vi "SimpleDemo old.vi"() -> ()   [LabVIEW 2011]
uses:
  C:/Users/Behavior Room/Desktop/Kinect Mouse/DepthSense/FunctionPointerProxy/FunctionPointerProxy/obj/Release/FunctionPointerProxy.dll
  FunctionPointerProxy/obj/Release/FunctionPointerProxy.dll
  <vilib>/vision/Image Controls.llb/IMAQ Image.ctl
  <vilib>/Platform/TimedLoop/XDataNode/timing_clust.ctl
  <vilib>/Platform/TimedLoop/XDataNode/nitl_modes.ctl
  <vilib>/Platform/TimedLoop/XDataNode/wakeup.ctl
  <vilib>/Platform/TimedLoop/XDataNode/XDataNode.xnode
  <userlib>/libOptrima-2-3/libOptrima-2-3.lvlib
  <vilib>/Platform/TimedLoop/XDataNode/XDNodeRunTimeDep.lvlib
  Program Files (x86)/SoftKinetic/OptrimaSDK/lib/libOptrima-2-3.dll
panel:
  out "length":i32
  out "add newframe\ncallback":i32
  in  "stop":bool
  in  "Buffer Size 3":i32=10
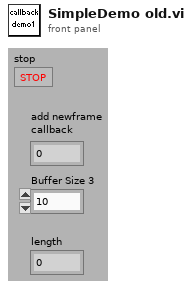
[diagram p1: front panel]
types:
  T1 = typedef "IMAQ Image.ctl" = refnum<image>
  T2 = typedef "XDNodeRunTimeDep.lvlib/timing_clust.ctl" = cluster{"Expected End [f-1]":u64, "Actual End [f-1]":u64, "Finished Late? [f-1]":bool, "Expected End [i-1]":u64, "Actual End [i-1]":u64, "Finished Late? [i-1]":bool, "Expected Start [i]":u64, "Actual Start [i]":u64, "Expected Start [f]":u64, "Actual Start [f]":u64, "Source Name":string, "Structure Name":string, "Period":i64, "Deadline":i64, "Offset":i64, "Start":i64, "Priority":i32, "Timeout":i32, "Mode":T3, "Wakeup Reason":T4, "Error":errorcluster, "Source Type":string, "Secondary Source Type":string, "Global End Time":u64, "Global Start Time":u64, "Frame Duration":u64, "Iteration Duration":u64, "Assigned CPU":i32, "I/O Scan Engine Mode":u32}
  T3 = typedef "XDNodeRunTimeDep.lvlib/nitl_modes.ctl" = enum32{"No Change", "Process missed periods, maintain original phase", "Discard missed periods, maintain original phase", "Process missed periods, ignore original phase", "Discard missed periods, ignore original phase"}
  T4 = typedef "XDNodeRunTimeDep.lvlib/wakeup.ctl" = enum32{"Normal", "Aborted", "Asynchronous wakeup", "Timing source error", "Timed loop error", "Timeout"}
  T5 = cluster{"queue out":refnum<queue>, "queue out":refnum<queue>}
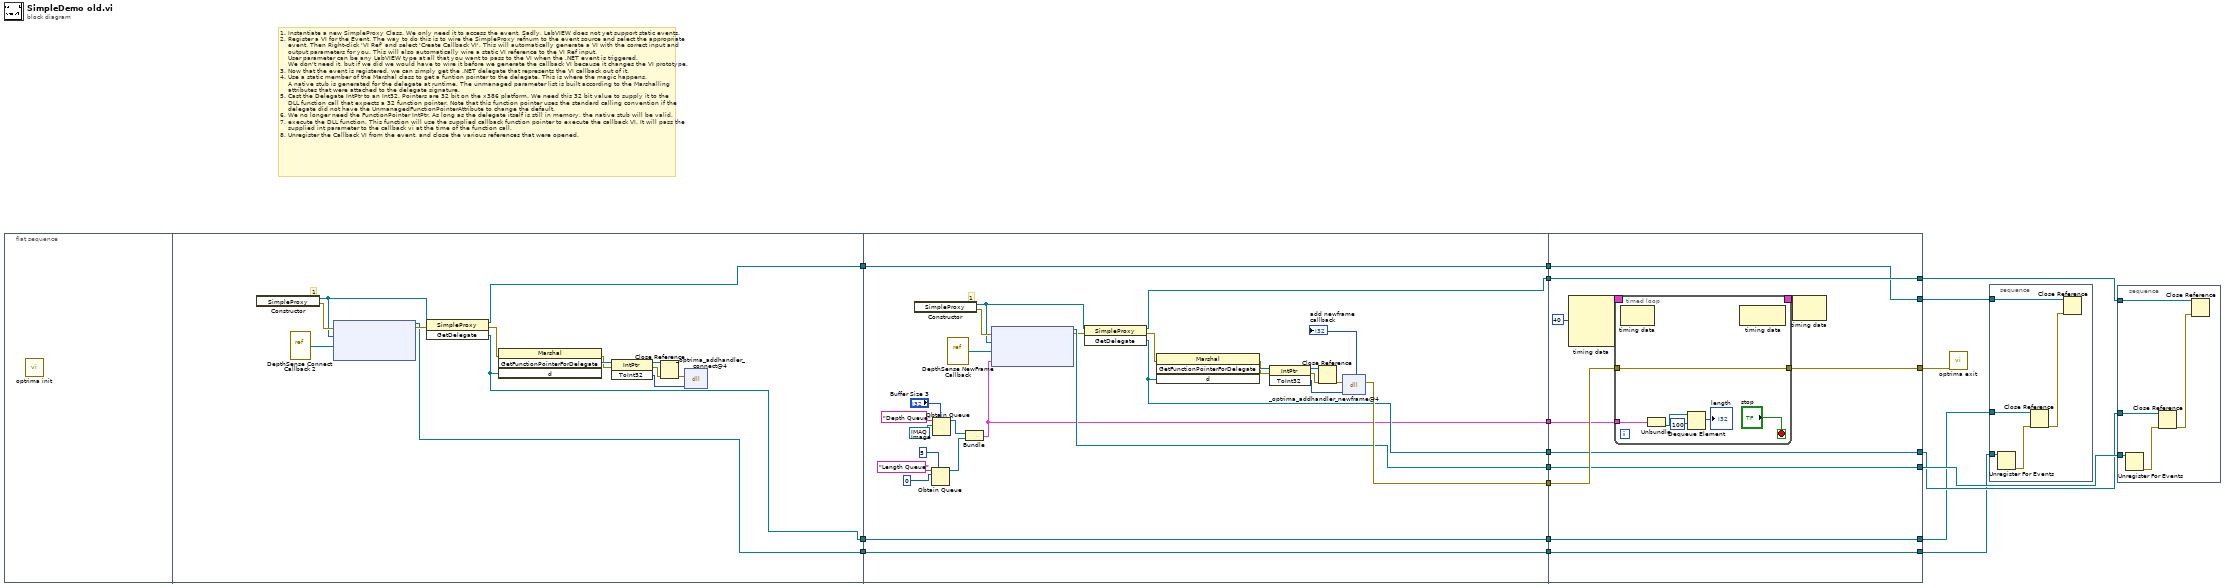
[diagram p0: block diagram]
diagram:
  # "1. Instantiate a new SimpleProxy Class. We only need it to access the event. Sadly, LabVIEW does not yet support static events.\n2. Register a VI for the Event. The way to do this is to wire the SimpleProxy refnum to the event source and select the appropriate\n    event. Then Right-click 'VI Ref' and select 'Create Callback VI'. This will automatically generate a VI with the correct input and\n    output parameters for you. This will also automatically wire a static VI reference to the VI Ref input.\n    User parameter can be any LabVIEW type at all that you want to pass to the VI when the .NET event is triggered.\n    We don't need it, but if we did we would have to wire it before we generate the callback VI because it changes the VI prototype.\n3. Now that the event is registered, we can simply get the .NET delegate that represents the VI callback out of it.\n4. Use a static member of the Marshal class to get a funtion pointer to the delegate. This is where the magic happens.\n    A native stub is generated for the delegate at runtime. The unmanaged parameter list is built according to the Marshalling\n    attributes that were attached to the delegate signature.\n5. Cast the Delegate IntPtr to an Int32. Pointers are 32 bit on the x386 platform. We need this 32 bit value to supply it to the\n    DLL function call that expects a 32 function pointer. Note that this function pointer uses the standard calling convention if the\n    delegate did not have the UnmanagedFunctionPointerAttribute to change the default.\n6. We no longer need the FunctionPointer IntPtr. As long as the delegate itself is still in memory, the native stub will be valid.\n7. execute the DLL function. This function will use the supplied callback function pointer to execute the callback VI. It will pass the\n    supplied int parameter to the callback vi at the time of the function call.\n8. Unregister the Callback VI from the event, and close the various references that were opened."
  n1 = flat-sequence {
    tunnel: [w21] -> w9
    tunnel: [w20] -> w6
    tunnel: [w19] -> w3
    tunnel: [w60] -> w18
    tunnel: [w59] -> w16
    tunnel: [w58] -> w14
    tunnel: [w57] -> w11
    tunnel: [w56] -> w10
    tunnel: w9 -> [w56]
    tunnel: w6 -> [w55]
    tunnel: [w55] -> w5
    tunnel: [w54] -> w4
    tunnel: w3 -> [w54]
    tunnel: [w34] -> w1
    tunnel: w18 -> [w72]
    tunnel: [w71] -> w17
    tunnel: [w67] -> w15
    tunnel: w16 -> [w67]
    tunnel: [w66] -> w13
    tunnel: w14 -> [w66]
    tunnel: [w65] -> w12
    tunnel: w11 -> [w65]
    tunnel: w10 -> [w64]
    tunnel: [w64] -> w8
    tunnel: [w63] -> w7
    tunnel: w5 -> [w63]
    tunnel: w4 -> [w62]
    tunnel: [w62] -> w2
    tunnel: w1 -> [w61]
    frame #0 {
      n2 = call <userlib>:"optrima init.vi"() -> ()  [unwired: 11 in, 1 out]
    }
    frame #1 {
      # "1"
      n3 = constructor class="SimpleProxy"() -> (reference out=w24:refnum<k24>, error out=w28:errorcluster)  [unwired: 3 in, 1 out]
      n4 = vi-ref "DepthSense Connect Callback 2.vi"() -> ("vi reference"=w22:refnum<vi>)
      n5 = node(w28, w24, w22) -> (w21:refnum<k27>, w32:errorcluster)  [unwired: 2 in]
      n6 = invoke class="SimpleProxy" method="GetDelegate"(reference=w24, error in=w32) -> (reference out=w19:refnum<k24>, error out=w30:errorcluster, "GetDelegate"=w20:refnum<k24>)  [unwired: 1 in]
      n7 = invoke class="Marshal" method="GetFunctionPointerForDelegate"(error in=w30, "d"=w20) -> (error out=w29:errorcluster, "GetFunctionPointerForDelegate"=w31:refnum<k24>)  [unwired: 2 in, 2 out]
      n8 = invoke class="IntPtr" method="ToInt32"(reference=w31, error in=w29) -> (reference out=w27:refnum<k24>, error out=w25:errorcluster, "ToInt32"=w23:i32)  [unwired: 1 in]
      n9 = Close Reference(reference=w27, error in (no error)=w25) -> (error out=w26:errorcluster)
      n10 = dll-call lib="C:/Program Files (x86)/SoftKinetic/OptrimaSDK/lib/libOptrima-2-3.dll" fn="_optrima_addhandler_connect@4"(error in=w26, "handlerfunc"=w23) -> ()  [unwired: 4 in, 2 out]
    }
    frame #2 {
      # "1"
      n11 = constructor class="SimpleProxy"() -> (reference out=w45:refnum<k24>, error out=w49:errorcluster)  [unwired: 3 in, 1 out]
      n12 = Obtain Queue(max queue size (-1, unlimited)=5, name (unnamed)="Length Queue", element data type=0) -> (queue out=w35:refnum<queue>)  [unwired: 2 in, 2 out]
      n13 = Obtain Queue(max queue size (-1, unlimited)="Buffer Size 3", name (unnamed)="Depth Queue", element data type=T1 refnum ("New Image")) -> (queue out=w39:refnum<queue>)  [unwired: 2 in, 2 out]
      n14 = vi-ref "DepthSense NewFrame Callback.vi"() -> ("vi reference"=w33:refnum<vi>)
      n15 = Bundle("queue out"=w39, "queue out"=w35) -> (w34:T5)  [unwired: 1 in]
      n16 = node(w49, w45, w33, w34) -> (w59:refnum<k27>, w53:errorcluster)  [unwired: 1 in]
      n17 = invoke class="SimpleProxy" method="GetDelegate"(reference=w45, error in=w53) -> (reference out=w57:refnum<k24>, error out=w51:errorcluster, "GetDelegate"=w58:refnum<k24>)  [unwired: 1 in]
      n18 = invoke class="Marshal" method="GetFunctionPointerForDelegate"(error in=w51, "d"=w58) -> (error out=w50:errorcluster, "GetFunctionPointerForDelegate"=w52:refnum<k24>)  [unwired: 2 in, 2 out]
      n19 = invoke class="IntPtr" method="ToInt32"(reference=w52, error in=w50) -> (reference out=w48:refnum<k24>, error out=w46:errorcluster, "ToInt32"=w44:i32)  [unwired: 1 in]
      n20 = Close Reference(reference=w48, error in (no error)=w46) -> (error out=w47:errorcluster)
      n21 = dll-call lib="C:/Program Files (x86)/SoftKinetic/OptrimaSDK/lib/libOptrima-2-3.dll" fn="_optrima_addhandler_newframe@4"(error in=w47, "handlerfunc"=w44) -> (error out=w60:errorcluster, "return type"=→"add newframe\ncallback":i32)  [unwired: 3 in, 1 out]
    }
    frame #3 {
      n22 = node-c288(i64 40 ("Period")) -> (w70:T2)  [unwired: 3 in]
      n23 = timed-loop {
        tunnel: [w77] -> w71
        tunnel: w72 -> [w77]
        timing: w70 -> [_]
        timing-out: [_] -> w69
        tunnel: w61 -> [w76]
        stop <- "stop" stop-if-true
        n24 = node-c288() -> ()  [unwired: 1 in, 1 out]
        n25 = Unbundle(w76) -> ("queue out"=w75:refnum<queue>)  [unwired: 1 out]
        n26 = Dequeue Element(queue=w75, timeout in ms (-1)=100) -> (element=→"length":i32)  [unwired: 1 in, 3 out]
        n27 = node-c288() -> ()  [unwired: 1 in, 1 out]
      }
      n28 = node-c288(w69) -> ()  [unwired: 1 out]
    }
  }
  n29 = call <userlib>:"optrima exit.vi"("error in (no error)"=w17) -> ()  [unwired: 10 in, 1 out]
  n30 = stacked-sequence {
    tunnel: w8 -> [w89]
    tunnel: w2 -> [w88]
    tunnel: w7 -> [w87]
    frame #0 {
      n31 = Unregister For Events(event registration refnum=w89) -> (error out=w86:errorcluster)  [unwired: 1 in]
      n32 = Close Reference(reference=w87, error in (no error)=w86) -> (error out=w85:errorcluster)
      n33 = Close Reference(reference=w88, error in (no error)=w85) -> ()  [unwired: 1 out]
    }
  }
  n34 = stacked-sequence {
    tunnel: w15 -> [w94]
    tunnel: w12 -> [w93]
    tunnel: w13 -> [w92]
    frame #0 {
      n35 = Unregister For Events(event registration refnum=w94) -> (error out=w91:errorcluster)  [unwired: 1 in]
      n36 = Close Reference(reference=w92, error in (no error)=w91) -> (error out=w90:errorcluster)
      n37 = Close Reference(reference=w93, error in (no error)=w90) -> ()  [unwired: 1 out]
    }
  }
